vi "get_status.vi"(1 "error in (no error)":errorcluster) -> (0 "error out":errorcluster)   [LabVIEW 2016]
uses:
  sa commands.ctl
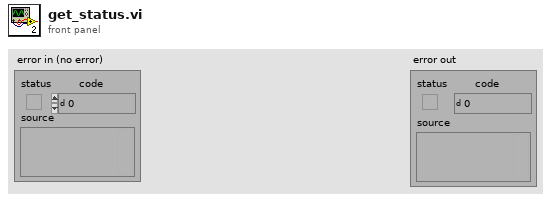
[diagram p1: front panel]
types:
  T1 = typedef "sa commands.ctl" = enum16{"read all", "set system index", "set x channel", "set y channel", "set rotation channel"}
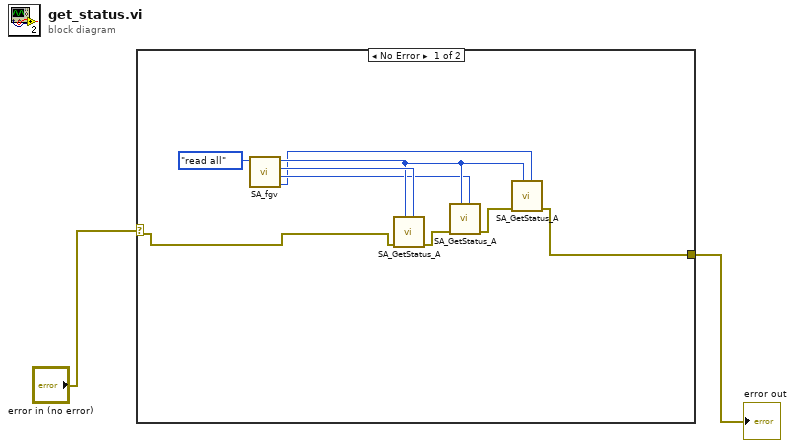
[diagram p0: block diagram]
diagram:
  n1 = case shown="No Error" "error in (no error)" {
    selector: "error in (no error)" -> [w10 w12]
    tunnel: [w6 w12] -> w1
    frame No Error {
      n2 = call "SA_fgv.vi"("command"=sa_commands."read all") -> ("rotation channel"=w3:u32, "y channel"=w4:u32, "x channel"=w9:u32, "system index"=w5:u32)  [unwired: 3 in]
      n3 = call <vilib>:"SA_GetStatus_A.vi"("channelIndex"=w9, "systemIndex"=w5, "error in (no error)"=w10) -> ("error out"=w8:errorcluster)  [unwired: 8 in]
      n4 = call <vilib>:"SA_GetStatus_A.vi"("channelIndex"=w4, "systemIndex"=w5, "error in (no error)"=w8) -> ("error out"=w7:errorcluster)  [unwired: 8 in]
      n5 = call <vilib>:"SA_GetStatus_A.vi"("channelIndex"=w3, "systemIndex"=w5, "error in (no error)"=w7) -> ("error out"=w6:errorcluster)  [unwired: 8 in]
    }
    frame Error {
    }
  }
  "error out" <- w1
